vi "Send Command.vi"(0 "reference in":refnum<class "NS master.lvclass">, 5 "message":string, 7 "parameters":string, 9 "data":variant, 11 "error in (no error)":errorcluster, 12 "response?":bool, 13 "timeout":i32=500) -> (4 "reference out":refnum<class "NS master.lvclass">, 6 "status":string, 8 "reponse":string, 10 "data":variant, 15 "error out":errorcluster)   [LabVIEW 2019, in "CommandResponse communication.lvlib" / "NS master.lvclass"]
doc: "Sends command as message + variant data and optionally awaits for response message and error"
uses:
  NS master.lvclass
  C:/Barkhausen mmWave radar/Development/LV/Barkhausen mmWave hardware control/Host/Intertarget communication/CR_master_class/CR_master.lvclass
  ITC command.ctl
  ITC response.ctl
  <userlib>/_OpenG.lib/string/string.llb/Trim Whitespace (String)__ogtk.vi
  CommandResponse communication.lvlib
  <resource>/objmgr/ni.dex.rc
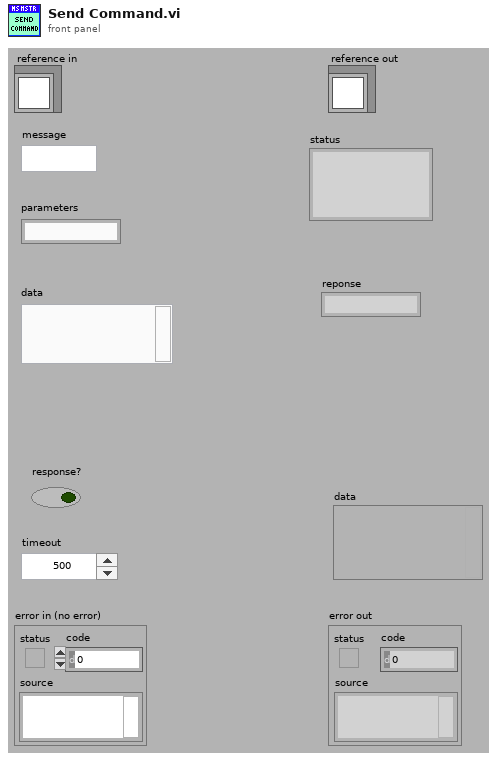
[diagram p1: front panel]
types:
  T1 = typedef "CommandResponse communication.lvlib/ITC command.ctl" = cluster{"message":string, "parameters":string, "data":variant}
  T2 = typedef "CommandResponse communication.lvlib/NS master.lvclass/ObjectAttributesRef.ctl" = refnum<data-value>
  T3 = typedef "CommandResponse communication.lvlib/NS master.lvclass/ObjectAttributes.ctl" = cluster{"connected":bool, "stop":bool, "ID":string, "command wr":refnum<k21>, "response rd":refnum<k21>, "data rd":refnum<k21>, "slave ip":string, "slave id":string}
  T4 = typedef "CommandResponse communication.lvlib/ITC response.ctl" = cluster{"status":string, "reponse":string, "data":variant}
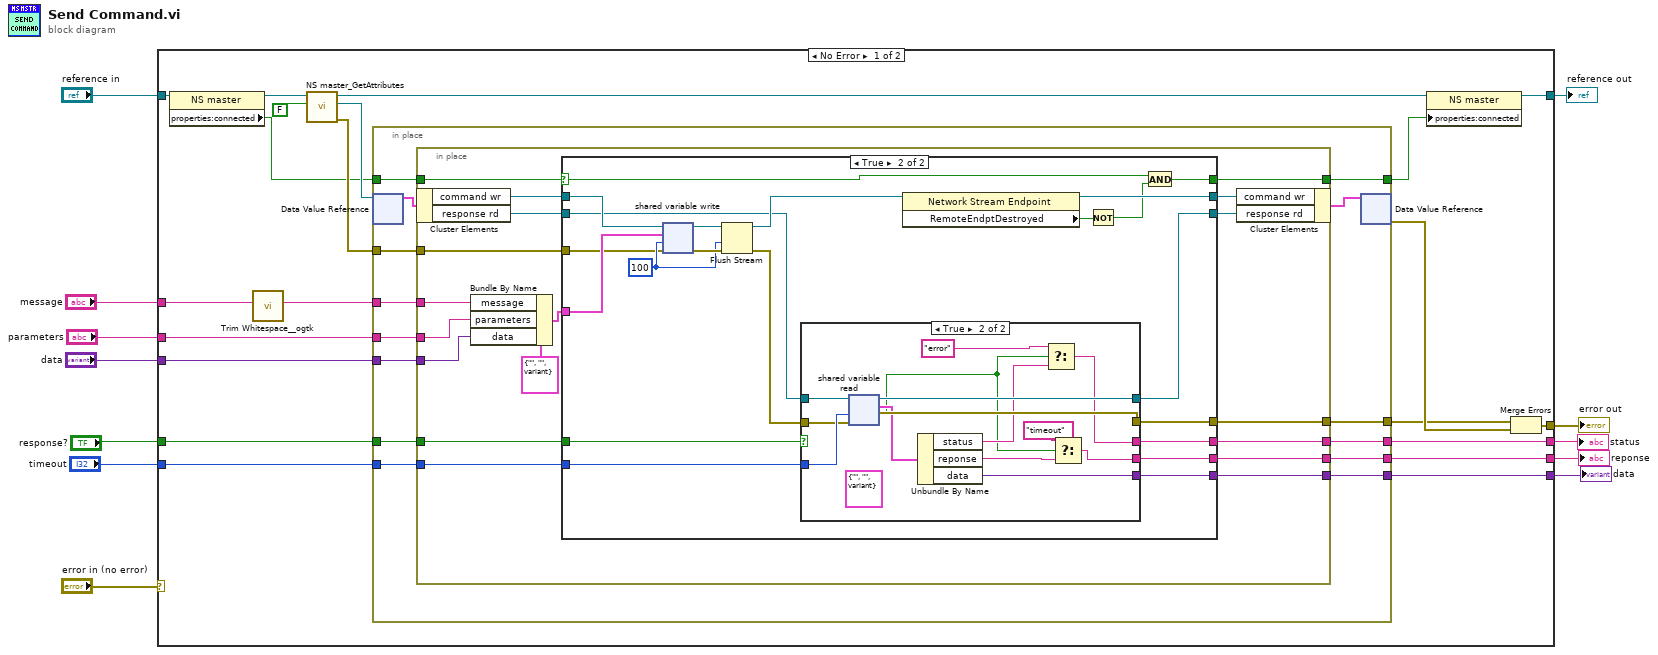
[diagram p0: block diagram]
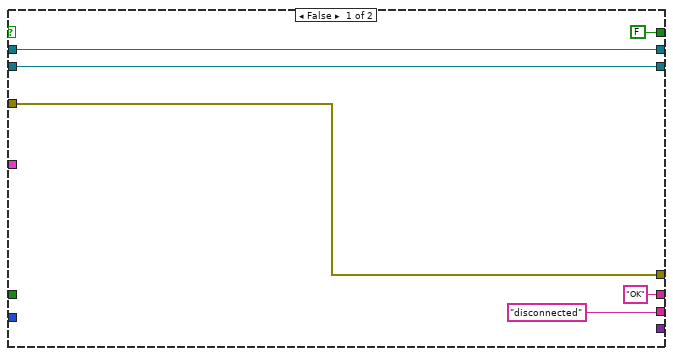
[diagram p2: hidden frame]
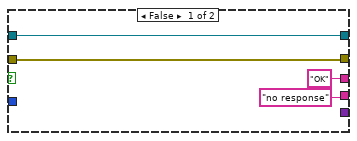
[diagram p3: hidden frame]
diagram:
  n1 = case shown="No Error" "error in (no error)" {
    selector: "error in (no error)" -> [_ w112]
    tunnel: [w33 w112] -> w11
    tunnel: [w15 w111] -> w9
    tunnel: "reference in" -> [w30 w111]
    tunnel: "message" -> [w26 _]
    tunnel: "parameters" -> [w25 _]
    tunnel: "response?" -> [w24 _]
    tunnel: "timeout" -> [w23 _]
    tunnel: [w21 _] -> w4
    tunnel: [w20 _] -> w3
    tunnel: [w19 _] -> w2
    tunnel: "data" -> [w18 _]
    frame No Error {
      n2 = property class="NS master"(reference=w30) -> (reference out=w17:refnum<class "NS master.lvclass">, "properties:connected"=w16:bool)  [unwired: 1 in, 1 out]
      n3 = call-poly <userlib>:"Trim Whitespace__ogtk.vi"("String in"=w26) -> ("String out"=w13:string)  [unwired: 6 in]
      n4 = call "NS master_GetAttributes.vi"("return data? (T)"=FALSE, "reference in"=w17) -> ("error out"=w22:errorcluster, "attributes ref"=w27:T2, "reference out"=w28:refnum<class "NS master.lvclass">)  [unwired: 6 in, 1 out]
      n5 = in-place {
        in-place-border: [w40] -> w31
        in-place-border: w13 -> [w45]
        in-place-border: w25 -> [w44]
        in-place-border: w24 -> [w43]
        in-place-border: w23 -> [w42]
        in-place-border: w22 -> [w41]
        in-place-border: [w39] -> w21
        in-place-border: [w38] -> w20
        in-place-border: [w37] -> w19
        in-place-border: w18 -> [w36]
        in-place-border: w16 -> [w35]
        in-place-border: [w34] -> w14
        n6 = in-place-dvr #1(w27) -> (w46:T3)  [unwired: 1 out]
        n7 = in-place {
          in-place-border: w45 -> [w61]
          in-place-border: w44 -> [w60]
          in-place-border: w43 -> [w57]
          in-place-border: w42 -> [w56]
          in-place-border: w41 -> [w55]
          in-place-border: [w54] -> w40
          in-place-border: [w53] -> w39
          in-place-border: [w52] -> w38
          in-place-border: [w51] -> w37
          in-place-border: w36 -> [w50]
          in-place-border: w35 -> [w49]
          in-place-border: [w48] -> w34
          n8 = in-place-cluster #2(w46) -> ("command wr"=w65:refnum<k21>, "response rd"=w59:refnum<k21>)
          n9 = Bundle By Name(cluster=T1 {"message"="", "parameters"="", "data"=variant} ("data in"), "message"=w61, "parameters"=w60, "data"=w50) -> (w62:T1)
          n10 = case shown="True" w49 {
            selector: w49 -> [_ w78]
            tunnel: w65 -> [w71 w90]
            tunnel: [w71 w75] -> w64
            tunnel: w62 -> [_ w88]
            tunnel: w59 -> [w70 w87]
            tunnel: [w70 w86] -> w58
            tunnel: w57 -> [_ w85]
            tunnel: w56 -> [_ w84]
            tunnel: w55 -> [w69 w81]
            tunnel: [w69 w80] -> w54
            tunnel: ["disconnected" ("status") w79] -> w53
            tunnel: [FALSE w73] -> w48
            tunnel: ["OK" ("status") w77] -> w52
            tunnel: [_ w76] -> w51
            frame False {
            }
            frame True {
              w83 = 100 ("timeout ms (-1)")
              n11 = shared-variable-write(w90, w81, w88, w83) -> (w92:refnum<k21>, w91:errorcluster)  [unwired: 1 out]
              n12 = Flush Stream(8:w91, 9:w83, 11:w92) -> (0:w82:errorcluster, 3:w89:refnum<k21>)  [unwired: 1 in, 1 out]
              n13 = case shown="True" w85 {
                tunnel: w87 -> [w96 w110]
                tunnel: [w96 w109] -> w86
                tunnel: w84 -> [_ w108]
                tunnel: w82 -> [w95 w107]
                tunnel: [w95 w106] -> w80
                tunnel: ["no response" ("reponse") w98] -> w79
                tunnel: ["OK" ("status") w101] -> w77
                tunnel: [_ w104] -> w76
                frame False {
                }
                frame True {
                  (unwired) T4 {"status"="", "reponse"="", "data"=variant} ("data out")
                  n14 = shared-variable-read(w110, w107, w108) -> (w109:refnum<k21>, w106:errorcluster, w100:bool, w105:T4)
                  n15 = Unbundle By Name(w105) -> ("status"=w103:string, "reponse"=w99:string, "data"=w104:variant)
                  n16 = Select(t="error", s=w100, f=w103) -> (s? t:f=w101:string)
                  n17 = Select(t="timeout", s=w100, f=w99) -> (s? t:f=w98:string)
                }
              }
              n18 = property class="Network Stream Endpoint"(reference=w89) -> (reference out=w75:refnum<k21>, "RemoteEndptDestroyed"=w74:bool)  [unwired: 1 in, 1 out]
              n19 = Not(x=w74) -> (.not. x?=w72:bool)
              n20 = And(x=w78, y=w72) -> (x .and. y?=w73:bool)
            }
          }
          n21 = in-place-cluster #2("command wr"=w64, "response rd"=w58) -> (w47:T3)
        }
        n22 = in-place-dvr #1(w47) -> (w32:errorcluster)  [unwired: 1 out]
      }
      n23 = property class="NS master"(reference=w28, "properties:connected"=w14) -> (reference out=w15:refnum<class "NS master.lvclass">)  [unwired: 1 in, 1 out]
      n24 = Merge Errors(w31, w32) -> (w33:errorcluster)
    }
    frame Error {
    }
  }
  "error out" <- w11
  "reference out" <- w9
  "reponse" <- w4
  "status" <- w3
  "data" <- w2
